vi "APG Return Configuration Directory.vi"() -> (2 "Configuration Directory":path)   [LabVIEW 2021]
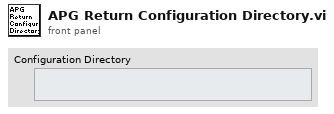
[diagram p1: front panel]
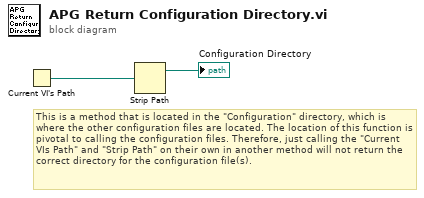
[diagram p0: block diagram]
diagram:
  # "This is a method that is located in the \"Configuration\" directory, which is where the other configuration files are located. The location of this function is pivotal to calling the configuration files. Therefore, just calling the \"Current VIs Path\" and \"Strip Path\" on their own in another method will not return the correct directory for the configuration file(s)."
  n1 = Current VI's Path() -> (path=w2:path)
  n2 = Strip Path(path=w2) -> (stripped path=→"Configuration Directory":path)  [unwired: 1 out]
